vi "Skip all.vi"(8 "error in (no error)":errorcluster, 11 "Run Block in":refnum<class "Run Block.lvclass">) -> (0 "error out":errorcluster, 3 "Run Block out":refnum<class "Run Block.lvclass">)   [LabVIEW 2020, in "CIRCUS_uServices.lvlib" / "Run Utilities.lvlib" / "Run Block.lvclass"]
doc: "Moves current RUN and all scripts from the schedule to skipped RUNs"
uses:
  Run Block.lvclass
  Run Instance/Run Instance.lvclass
  Schedule/Schedule.lvclass
  Cell/Schedule Cell.lvclass
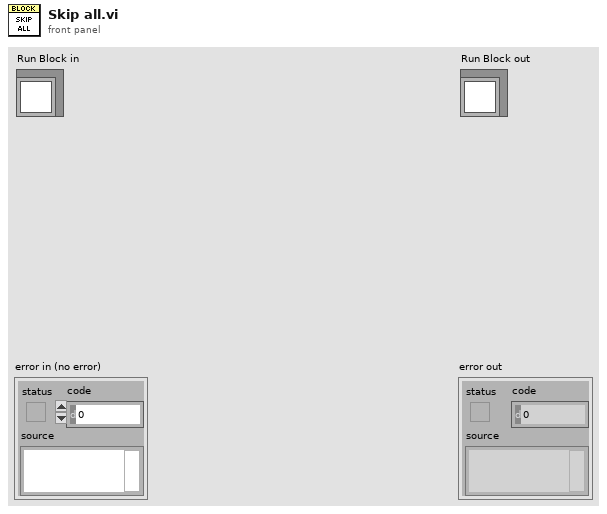
[diagram p1: front panel]
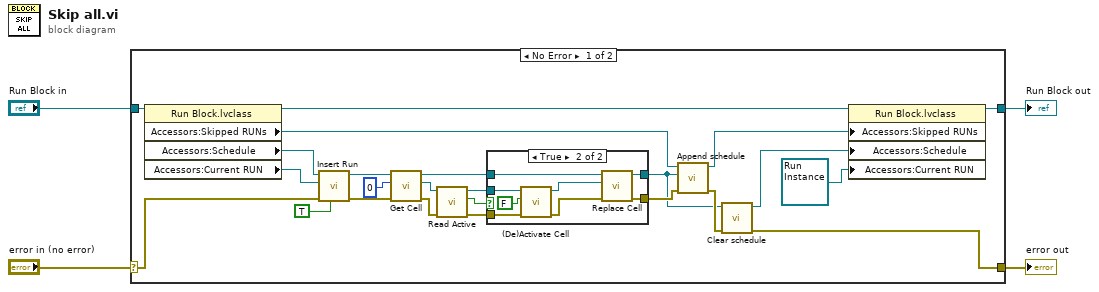
[diagram p0: block diagram]
diagram:
  n1 = case shown="No Error" "error in (no error)" {
    selector: "error in (no error)" -> [w17 w40]
    tunnel: [w20 w40] -> w3
    tunnel: [w25 w39] -> w1
    tunnel: "Run Block in" -> [w27 w39]
    frame No Error {
      n2 = property class="Run Block.lvclass"(reference=w27) -> (reference out=w26:refnum<class "Run Block.lvclass">, "Accessors:Skipped RUNs"=w24:refnum<class "Schedule.lvclass">, "Accessors:Schedule"=w19:refnum<class "Schedule.lvclass">, "Accessors:Current RUN"=w18:refnum<class "Run Instance.lvclass">)  [unwired: 1 in, 1 out]
      n3 = call-dynamic "Insert Run.vi"("Reinsert?"=TRUE, "error in (no error)"=w17, "Run Instance"=w18, "Schedule in"=w19) -> ("error out"=w13:errorcluster, "Schedule out"=w14:refnum<class "Schedule.lvclass">)  [unwired: 5 in, 1 out]
      n4 = call-dynamic "Get Cell.vi"("error in (no error)"=w13, "index"=0, "Schedule in"=w14) -> ("error out"=w11:errorcluster, "Schedule Cell"=w12:refnum<class "Schedule Cell.lvclass">, "Schedule out"=w7:refnum<class "Schedule.lvclass">)  [unwired: 6 in]
      n5 = call-dynamic "Read Active.vi"("error in (no error)"=w11, "Schedule Cell in"=w12) -> ("error out"=w10:errorcluster, "Active"=w9:bool, "Schedule Cell out"=w8:refnum<class "Schedule Cell.lvclass">)  [unwired: 7 in]
      n6 = case shown="True" w9 {
        tunnel: w8 -> [_ w38]
        tunnel: w10 -> [w29 w37]
        tunnel: w7 -> [w30 w35]
        tunnel: [w30 w34] -> w6
        tunnel: [w29 w33] -> w28
        frame False {
        }
        frame True {
          n7 = call-dynamic "(De)Activate Cell.vi"("error in (no error)"=w37, "Active"=FALSE, "Schedule Cell in"=w38) -> ("error out"=w32:errorcluster, "Schedule Cell out"=w31:refnum<class "Schedule Cell.lvclass">)  [unwired: 7 in]
          n8 = call-dynamic "Replace Cell.vi"("error in (no error)"=w32, "Schedule Cell"=w31, "Schedule in"=w35) -> ("error out"=w33:errorcluster, "Schedule out"=w34:refnum<class "Schedule.lvclass">)  [unwired: 7 in]
        }
      }
      n9 = call-dynamic "Append schedule.vi"("error in (no error)"=w28, "Schedule to append"=w6, "Schedule in"=w24) -> ("error out"=w22:errorcluster, "Schedule out"=w23:refnum<class "Schedule.lvclass">)  [unwired: 7 in]
      n10 = call-dynamic "Clear schedule.vi"("error in (no error)"=w22, "Schedule in"=w6) -> ("error out"=w20:errorcluster, "Schedule out"=w21:refnum<class "Schedule.lvclass">)  [unwired: 8 in]
      n11 = property class="Run Block.lvclass"(reference=w26, "Accessors:Skipped RUNs"=w23, "Accessors:Schedule"=w21, "Accessors:Current RUN"=refnum<class "Run Instance.lvclass"> refnum ("Current RUN")) -> (reference out=w25:refnum<class "Run Block.lvclass">)  [unwired: 1 in, 1 out]
    }
    frame Error {
    }
  }
  "error out" <- w3
  "Run Block out" <- w1
